vi "Update From Actor Ref FGV.vi"(8 "error in (no error)":errorcluster, 11 "Debugger in":refnum<class "Debugger.lvclass">) -> (0 "error out":errorcluster, 3 "Debugger out":refnum<class "Debugger.lvclass">)   [LabVIEW 2015, in "Debugger.lvclass"]
uses:
  Debugger.lvclass
  Debug Tools/Actor Ref Cache/Actor Ref Cache Action.ctl
  Debugger.lvclass/Debugger.ctl
  Utility/Utility.lvlib
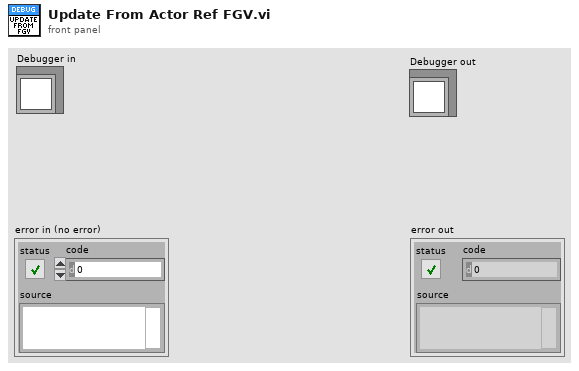
[diagram p1: front panel]
types:
  T1 = typedef "Actor Ref Cache Action.ctl" = enum16{"Clear", "Add Ref", "Remove Ref", "Get All Refs"}
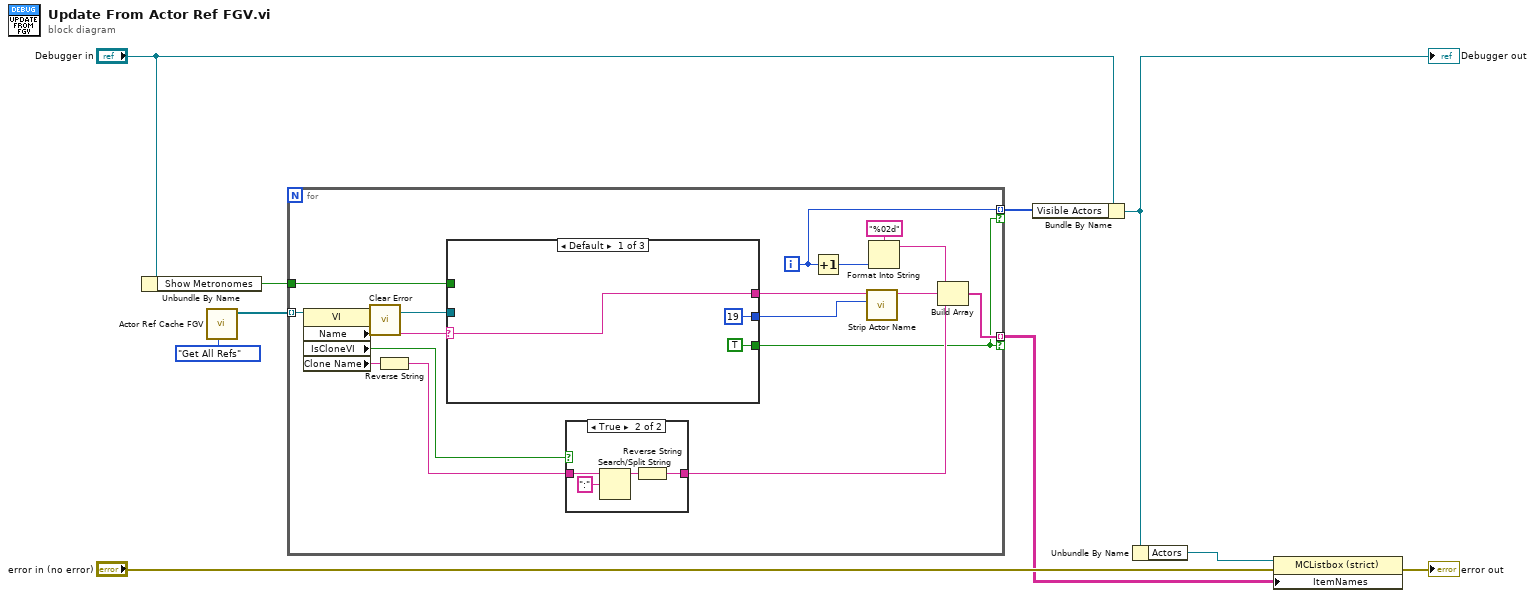
[diagram p0: block diagram]
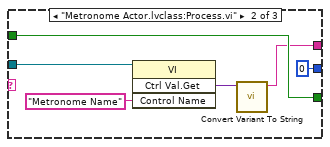
[diagram p2: hidden frame]
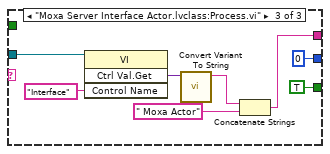
[diagram p3: hidden frame]
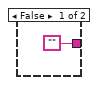
[diagram p4: hidden frame]
diagram:
  n1 = Unbundle By Name("Debugger in") -> ("Show Metronomes"=w10:bool)
  n2 = call "Actor Ref Cache FGV.vi"("Action"=Actor_Ref_Cache_Action."Get All Refs") -> ("All Refs Out"=w7:refnum<vi>[])  [unwired: 10 in]
  n3 = for {
    tunnel: w7 -> [w28] mode=indexing
    tunnel: [w26] -> w2 mode=indexing if=w11
    tunnel: w10 -> [w19]
    tunnel: [w12] -> w1 mode=indexing if=w11
    i -> [w12]
    n4 = property class="VI"(reference=w28) -> (reference out=w18:refnum<vi>, error out=w27:errorcluster, "Name"=w20:string, "IsCloneVI"=w23:bool, "Clone Name"=w24:string)  [unwired: 1 in]
    n5 = call "Clear Error.vi"("error in (no error)"=w27) -> ()  [unwired: 1 out]
    n6 = Reverse String(1:w24) -> (0:w25:string)
    n7 = case shown="Default" w20 {
      selector: w20 -> [w31 _ _]
      tunnel: [w31 w33 w39] -> w14
      tunnel: w19 -> [_ w37 _]
      tunnel: [TRUE w37 TRUE ("Show Clones")] -> w11
      tunnel: w18 -> [_ w36 w45]
      tunnel: [19 0 0] -> w16
      frame Default {
      }
      frame "Metronome Actor.lvclass:Process.vi" {
        n8 = invoke class="VI" method="Ctrl Val.Get"(reference=w36, "Control Name"="Metronome Name") -> ("Get Control Value Variant"=w34:variant)  [unwired: 2 in, 3 out]
        n9 = call "Convert Variant To String.vi"("Variant"=w34) -> ("String"=w33:string)  [unwired: 9 in, 1 out]
      }
      frame "Moxa Server Interface Actor.lvclass:Process.vi" {
        n10 = invoke class="VI" method="Ctrl Val.Get"(reference=w45, "Control Name"="Interface") -> ("Get Control Value Variant"=w43:variant)  [unwired: 2 in, 3 out]
        n11 = call "Convert Variant To String.vi"("Variant"=w43) -> ("String"=w41:string)  [unwired: 9 in, 1 out]
        n12 = Concatenate Strings(w41, " Moxa Actor" ("string")) -> (w39:string)
      }
    }
    n13 = case shown="True" w23 {
      tunnel: ["" w47] -> w13
      tunnel: w25 -> [_ w50]
      frame False {
      }
      frame True {
        n14 = Search/Split String(string=w50, search string/char (-)=":") -> (substring before match=w48:string)  [unwired: 1 in, 2 out]
        n15 = Reverse String(1:w48) -> (0:w47:string)
      }
    }
    n16 = Increment(x=w12) -> (x+1=w21:i32)
    n17 = call "Strip Actor Name.vi"("Characters From End To Strip"=w16, "Actor Name in"=w14) -> ("Actor Name out"=w17:string)  [unwired: 9 in]
    n18 = Format Into String(format string="%02d", w21) -> (resulting string=w15:string)  [unwired: 2 in, 1 out]
    n19 = Build Array(w15, w17, w13) -> (w26:string[])
  }
  n20 = Bundle By Name(cluster="Debugger in", "Visible Actors"=w1) -> (w6:refnum<class "Debugger.lvclass">)
  "Debugger out" <- w6
  n21 = Unbundle By Name(w6) -> ("Actors"=w5:refnum<vi>)
  n22 = property on="Property Node" class="MCListbox (strict)"(reference=w5, error in="error in (no error)", "ItemNames"=w2) -> (error out=→"error out":errorcluster)  [unwired: 1 out]
